vi "ChoosePanel.vi"() -> ()   [LabVIEW 2015]
uses:
  Fin_GlobalPath.vi
  Fin_GlobalData.vi
  Fin_GlobalVi.vi
panel:
  out "Panel Type":string
  out "Log File extension":string
  in  "Create log file?":bool
  in  "Done ?":bool
  in  "String 2":string
  in  "String":string
  # "Creating a log file"
  # "R"
  # "S1-0000-00"
  # "(in the first field add \"S\" for stereo and \"E\" for eta panel e.g. RSE1-0000-0005)"
  # "Panel name:"
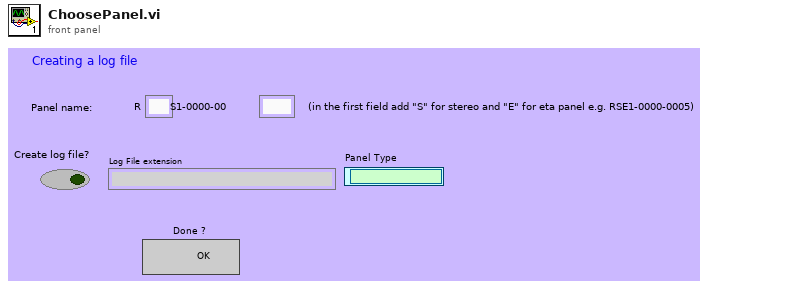
[diagram p1: front panel]
types:
  T1 = enum16{"open", "replace", "create", "open or create", "replace or create", "replace or create with confirmation"}
  T2 = enum32{"Bad", "Idle", "Run top level", "Running"}
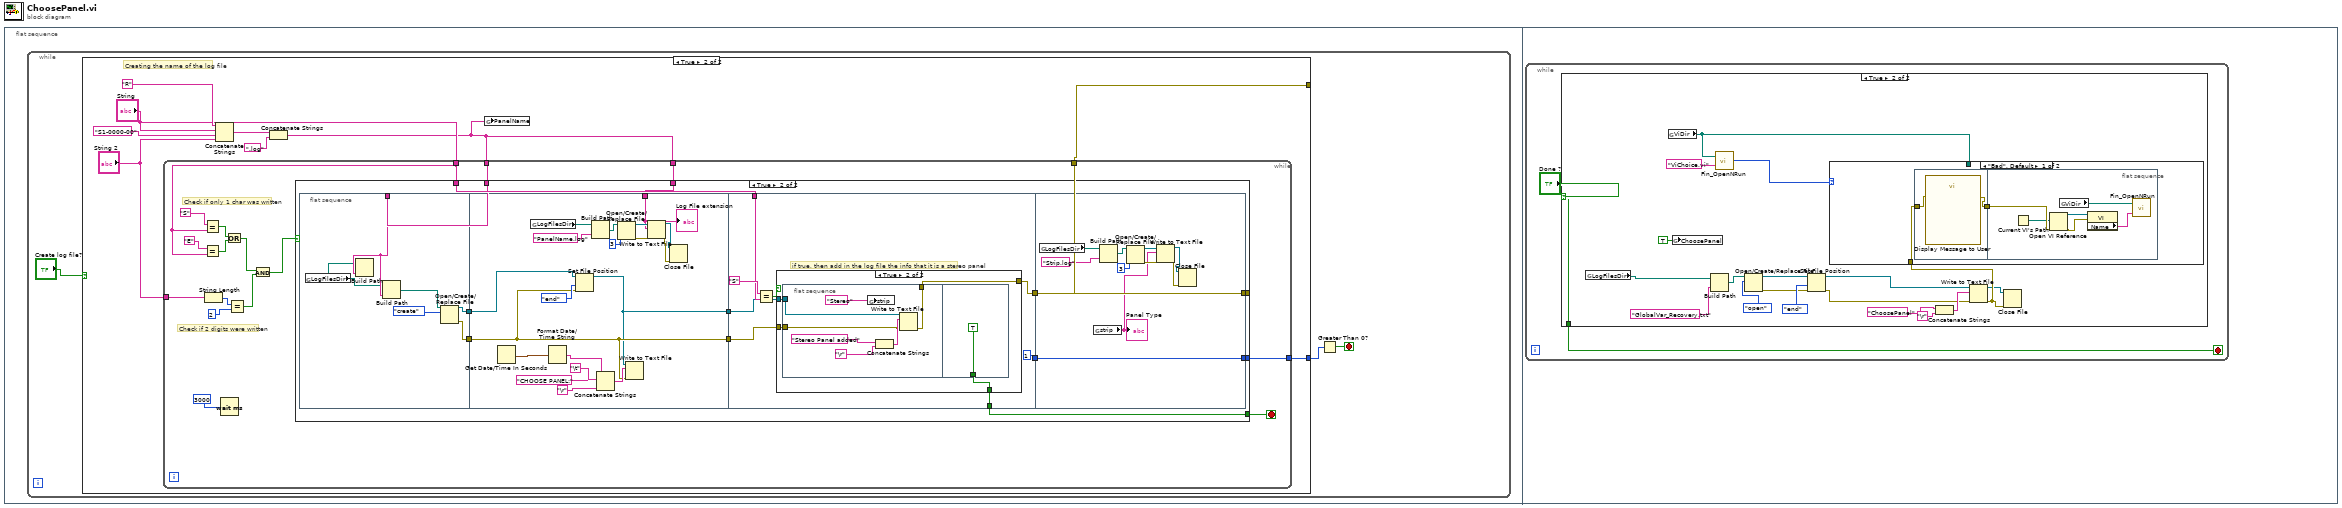
[diagram p0: block diagram]
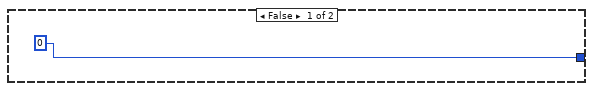
[diagram p2: hidden frame]
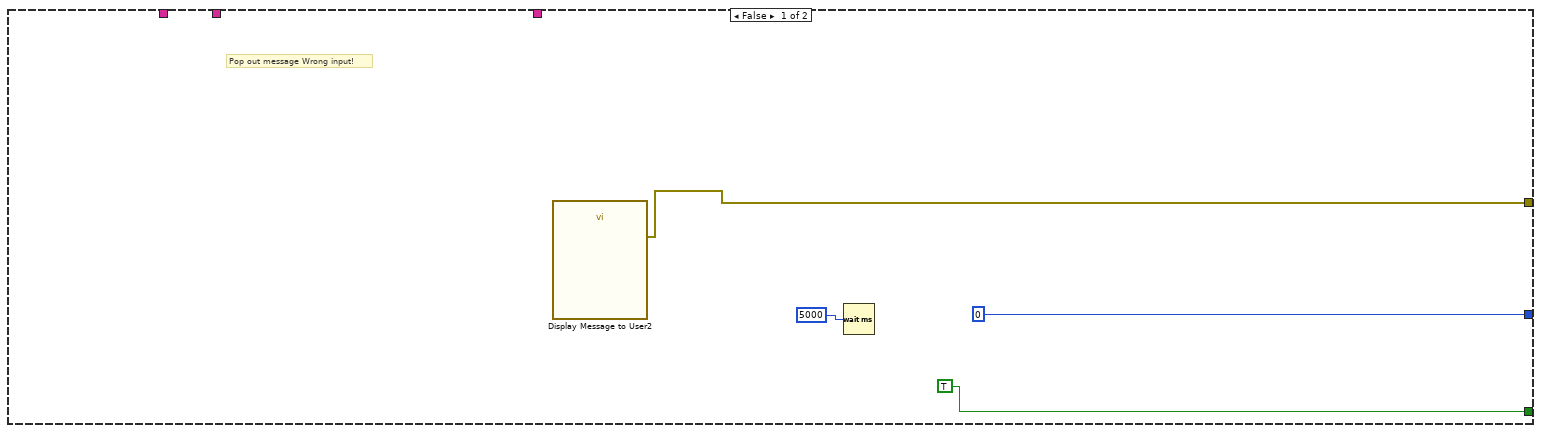
[diagram p3: hidden frame]
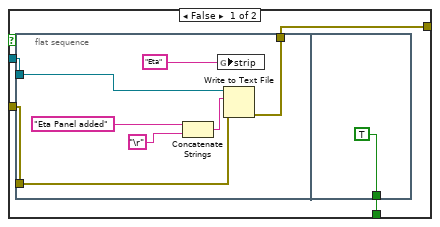
[diagram p4: hidden frame]
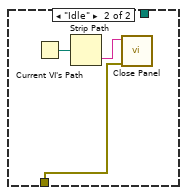
[diagram p6: hidden frame]
diagram:
  n1 = flat-sequence {
    frame #0 {
      n2 = while {
        stop <- w3 stop-if-true
        n3 = case shown="True" "Create log file?" {
          tunnel: [0 w8] -> w2
          tunnel: [_ w7] -> _
          frame False {
          }
          frame True {
            # "Creating the name of the log file"
            n4 = Concatenate Strings("R", "String", "S1-0000-00", "String 2") -> (w6:string)
            n5 = Concatenate Strings(w6, ".log") -> (w5:string)
            n6 = while {
              tunnel: "String" -> [w29]
              tunnel: w5 -> [w25]
              tunnel: "String 2" -> [w23]
              tunnel: [w17] -> w7
              tunnel: [w16] -> w8
              tunnel: w5 -> [w14]
              stop <- w24 stop-if-true
              # "Check if 2 digits were written"
              # "Check if only 1 char was written"
              n7 = Equal?(x="S", y=w29) -> (x = y?=w27:bool)
              n8 = Equal?(x="E", y=w29) -> (x = y?=w26:bool)
              n9 = String Length(string=w23) -> (length=w22:i32)
              n10 = Wait (ms)(milliseconds to wait=3000) -> ()  [unwired: 1 out]
              n11 = Or(x=w27, y=w26) -> (x .or. y?=w19:bool)
              n12 = Equal?(x=w22, y=2) -> (x = y?=w20:bool)
              n13 = And(x=w19, y=w20) -> (x .and. y?=w18:bool)
              n14 = case shown="True" w18 {
                tunnel: w29 -> [_ w46]
                tunnel: w25 -> [_ w38]
                tunnel: [TRUE w45] -> w24
                tunnel: [w33 w44] -> w17
                tunnel: [0 w39] -> w16
                tunnel: w14 -> [_ w37]
                frame False {
                  # "Pop out message Wrong input!"
                  n15 = call "Display Message to User2"() -> ("error out"=w33:errorcluster)  [unwired: 10 in, 1 out]
                  n16 = Wait (ms)(milliseconds to wait=5000) -> ()  [unwired: 1 out]
                }
                frame True {
                  n17 = flat-sequence {
                    tunnel: w38 -> [w48]
                    tunnel: [w49] -> w43
                    tunnel: [w51] -> w41
                    tunnel: w43 -> [w64]
                    tunnel: [w63] -> w42
                    tunnel: w41 -> [w65]
                    tunnel: [w65] -> w40
                    tunnel: w37 -> [w55]
                    tunnel: w46 -> [w77]
                    tunnel: w42 -> [w76]
                    tunnel: [w75] -> w45
                    tunnel: w40 -> [w74]
                    tunnel: [w73] -> w36
                    tunnel: [1] -> w35
                    tunnel: [w113] -> w39
                    tunnel: [w114] -> w44
                    tunnel: w36 -> [w114]
                    tunnel: w35 -> [w113]
                    frame #0 {
                      n18 = global read "Fin_GlobalPath.vi" "LogFilesDir"() -> (w47:path)
                      n19 = Build Path(base path=w47, name or relative path=w48) -> ()  [unwired: 1 out]
                      n20 = Build Path(base path=w47, name or relative path=w48) -> (appended path=w52:path)
                      n21 = Open/Create/Replace File(file path (use dialog)=w52, operation (0:open)=T1."create") -> (refnum out=w49:refnum<file>, error out=w51:errorcluster)  [unwired: 4 in, 1 out]
                    }
                    frame #1 {
                      n22 = Get Date/Time In Seconds() -> (seconds since 1Jan1904=w62:timestamp)
                      n23 = global read "Fin_GlobalPath.vi" "LogFilesDir"() -> (w56:path)
                      n24 = Format Date/Time String(seconds (now)=w62) -> (date/time string=w69:string)  [unwired: 2 in]
                      n25 = Set File Position(refnum=w64, from (0:start)=enum16{"start", "end", "current"}."end", error in=w65) -> (refnum out=w63:refnum<file>)  [unwired: 1 in, 1 out]
                      n26 = Build Path(base path=w56, name or relative path="PanelName.log") -> (appended path=w58:path)
                      n27 = Concatenate Strings(w69, "\t", "CHOOSE PANEL:", "\r") -> (w67:string)
                      n28 = Open/Create/Replace File(file path (use dialog)=w58, operation (0:open)=3) -> (refnum out=w61:refnum<file>, error out=w60:errorcluster)  [unwired: 4 in, 1 out]
                      n29 = Write to Text File(file (use dialog)=w63, text=w67, error in=w65) -> ()  [unwired: 1 in, 3 out]
                      n30 = Write to Text File(file (use dialog)=w61, text=w55, error in=w60) -> (refnum out=w54:refnum<file>, error out=w53:errorcluster)  [unwired: 1 in, 1 out]
                      n31 = Close File(refnum=w54, error in=w53) -> ()  [unwired: 2 out]
                      "Log File extension" <- w55
                    }
                    frame #2 {
                      # "if true, then add in the log file the info that it is a stereo panel"
                      n32 = Equal?(x="S", y=w77) -> (x = y?=w79:bool)
                      n33 = case shown="True" w79 {
                        tunnel: w76 -> [w83 w95]
                        tunnel: [w82 w94] -> w75
                        tunnel: w74 -> [w81 w93]
                        tunnel: [w80 w92] -> w73
                        frame False {
                          n34 = flat-sequence {
                            tunnel: w83 -> [w90]
                            tunnel: w81 -> [w87]
                            tunnel: [w86] -> w80
                            tunnel: [TRUE] -> w82
                            frame #0 {
                              n35 = Concatenate Strings("Eta Panel added", "\r") -> (w89:string)
                              n36 = global write "Fin_GlobalData.vi" "strip"("Eta") -> ()
                              n37 = Write to Text File(file (use dialog)=w90, text=w89, error in=w87) -> (error out=w86:errorcluster)  [unwired: 1 in, 2 out]
                            }
                            frame #1 {
                            }
                          }
                        }
                        frame True {
                          n38 = flat-sequence {
                            tunnel: w95 -> [w102]
                            tunnel: w93 -> [w99]
                            tunnel: [w98] -> w92
                            tunnel: [TRUE] -> w94
                            frame #0 {
                              n39 = global write "Fin_GlobalData.vi" "strip"("Stereo") -> ()
                              n40 = Concatenate Strings("Stereo Panel added", "\r") -> (w101:string)
                              n41 = Write to Text File(file (use dialog)=w102, text=w101, error in=w99) -> (error out=w98:errorcluster)  [unwired: 1 in, 2 out]
                            }
                            frame #1 {
                            }
                          }
                        }
                      }
                    }
                    frame #3 {
                      n42 = global read "Fin_GlobalPath.vi" "LogFilesDir"() -> (w107:path)
                      n43 = global read "Fin_GlobalData.vi" "strip"() -> (w104:string)
                      "Panel Type" <- w104
                      n44 = Build Path(base path=w107, name or relative path="Strip.log") -> (appended path=w109:path)
                      n45 = Open/Create/Replace File(file path (use dialog)=w109, operation (0:open)=3) -> (refnum out=w112:refnum<file>, error out=w111:errorcluster)  [unwired: 4 in, 1 out]
                      n46 = Write to Text File(file (use dialog)=w112, text=w104, error in=w111) -> (refnum out=w106:refnum<file>, error out=w105:errorcluster)  [unwired: 1 in, 1 out]
                      n47 = Close File(refnum=w106, error in=w105) -> ()  [unwired: 2 out]
                    }
                  }
                }
              }
            }
            n48 = global write "Fin_GlobalData.vi" "PanelName"(w5) -> ()
          }
        }
        n49 = Greater Than 0?(x=w2) -> (x > 0?=w3:bool)
      }
    }
    frame #1 {
      n50 = while {
        stop <- w115 stop-if-true
        n51 = case shown="True" "Done ?" {
          selector: "Done ?" -> [w117 w133]
          tunnel: [w117 w133] -> w115
          frame False {
          }
          frame True {
            n52 = global read "Fin_GlobalPath.vi" "LogFilesDir"() -> (w121:path)
            n53 = global read "Fin_GlobalPath.vi" "ViDir"() -> (w134:path)
            n54 = global write "Fin_GlobalVi.vi" "ChoosePanel"(TRUE) -> ()
            n55 = Build Path(base path=w121, name or relative path="GlobalVar_Recovery.txt") -> (appended path=w131:path)
            n56 = call "Fin_OpenNRun.vi"("VI name"="ViChoice.vi", "ViDirPath"=w134) -> ("Execution:State"=w136:T2)
            n57 = Open/Create/Replace File(file path (use dialog)=w131, operation (0:open)=T1."open") -> (refnum out=w127:refnum<file>, error out=w128:errorcluster)  [unwired: 4 in, 1 out]
            n58 = Set File Position(refnum=w127, from (0:start)=enum16{"start", "end", "current"}."end", error in=w128) -> (refnum out=w124:refnum<file>, error out=w123:errorcluster)  [unwired: 1 in]
            n59 = Concatenate Strings("ChoosePanel", "\r") -> (w126:string)
            n60 = Write to Text File(file (use dialog)=w124, text=w126, error in=w123) -> (refnum out=w119:refnum<file>, error out=w120:errorcluster)  [unwired: 1 in, 1 out]
            n61 = case shown="\"Bad\", Default" w136 {
              tunnel: w134 -> [_ _]
              tunnel: w120 -> [w137 w147]
              frame "Bad", Default {
                n62 = flat-sequence {
                  tunnel: w137 -> [w140]
                  tunnel: [w139] -> w138
                  tunnel: w138 -> [w143]
                  frame #0 {
                    n63 = call "Display Message to User"("error in (no error)"=w140) -> ("error out"=w139:errorcluster)  [unwired: 9 in, 1 out]
                  }
                  frame #1 {
                    n64 = Current VI's Path() -> (path=w141:path)
                    n65 = Open VI Reference(vi path=w141, error in (no error)=w143) -> (vi reference=w146:refnum<vi>, error out=w145:errorcluster)  [unwired: 4 in]
                    n66 = global read "Fin_GlobalPath.vi" "ViDir"() -> (w142:path)
                    n67 = property class="VI"(reference=w146, error in=w145) -> ("Name"=w144:string)  [unwired: 2 out]
                    n68 = call "Fin_OpenNRun.vi"("VI name"=w144, "ViDirPath"=w142) -> ()  [unwired: 1 out]
                  }
                }
              }
              frame "Idle" {
                n69 = Current VI's Path() -> (path=w148:path)
                n70 = Strip Path(path=w148) -> (name=w149:string)  [unwired: 1 out]
                n71 = call <vilib>:"Close Panel.vi"("error in (no error)"=w147, "VI name"=w149) -> ()  [unwired: 9 in, 1 out]
              }
            }
            n72 = Close File(refnum=w119, error in=w120) -> ()  [unwired: 2 out]
          }
        }
      }
    }
  }
